vi "Analog Trigger.vi"() -> ()   [LabVIEW 2012]
uses:
  <vilib>/Platform/TimedLoop/XDataNode/timing_clust.ctl
  <vilib>/Platform/TimedLoop/XDataNode/nitl_modes.ctl
  <vilib>/Platform/TimedLoop/XDataNode/wakeup.ctl
  <vilib>/rvi/eio/common/nirviEmuTemplateMethod_errors.vi
  <vilib>/rvi/Emulation/niFpgaSctlEmulationRegisterWithScheduler.vi
  <vilib>/rvi/Emulation/niFpgaSctlEmulationScheduler.vi
  <vilib>/Platform/TimedLoop/XDataNode/XDataNode.xnode
  <vilib>/eio/EIONode/EIONode.xnode
  <vilib>/Platform/TimedLoop/XDataNode/XDNodeRunTimeDep.lvlib
panel:
  out "Over Threshold":bool
  in  "stop":bool
  in  "Threshold":i16
  out "AI Ch 0":i16
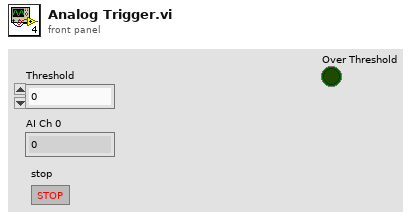
[diagram p1: front panel]
types:
  T1 = typedef "XDNodeRunTimeDep.lvlib/timing_clust.ctl" = cluster{"Expected End [f-1]":u64, "Actual End [f-1]":u64, "Finished Late? [f-1]":bool, "Expected End [i-1]":u64, "Actual End [i-1]":u64, "Finished Late? [i-1]":bool, "Expected Start [i]":u64, "Actual Start [i]":u64, "Expected Start [f]":u64, "Actual Start [f]":u64, "Source Name":string, "Structure Name":string, "Period":i64, "Deadline":i64, "Offset":i64, "Start":i64, "Priority":i32, "Timeout":i32, "Mode":T2, "Wakeup Reason":T3, "Error":errorcluster, "Source Type":string, "Secondary Source Type":string, "Global End Time":u64, "Global Start Time":u64, "Frame Duration":u64, "Iteration Duration":u64, "Assigned CPU":i32, "I/O Scan Engine Mode":u32}
  T2 = typedef "XDNodeRunTimeDep.lvlib/nitl_modes.ctl" = enum32{"No Change", "Process missed periods, maintain original phase", "Discard missed periods, maintain original phase", "Process missed periods, ignore original phase", "Discard missed periods, ignore original phase"}
  T3 = typedef "XDNodeRunTimeDep.lvlib/wakeup.ctl" = enum32{"Normal", "Aborted", "Asynchronous wakeup", "Timing source error", "Timed loop error", "Timeout"}
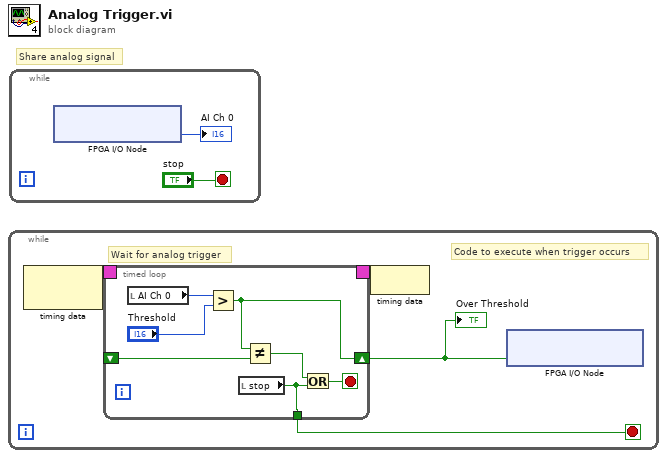
[diagram p0: block diagram]
diagram:
  # "Share analog signal"
  n1 = while {
    stop <- w1 stop-if-true
    # "Code to execute when trigger occurs"
    # "Wait for analog trigger"
    n2 = node-c288() -> (w4:T1)  [unwired: 1 in]
    n3 = timed-loop {
      timing: w4 -> [_]
      timing-out: [_] -> w3
      shift-right: [w9] -> w2
      shift-left: _ -> [w8]
      tunnel: [w5] -> w1
      stop <- w6 stop-if-true
      n4 = local read "AI Ch 0"() -> (w11:i16)
      n5 = Greater?(x=w11, y="Threshold") -> (0:w9:bool)
      n6 = local read "stop"() -> (w5:bool)
      n7 = Not Equal?(x=w9, y=w8) -> (x != y?=w7:bool)
      n8 = Or(x=w7, y=w5) -> (x .or. y?=w6:bool)
    }
    "Over Threshold" <- w2
    n9 = node-c288(w3) -> ()
    n10 = xnode "FPGA I/O Node"("Connector0/DIO0"=w2) -> ()  [unwired: 1 in, 1 out]
  }
  n11 = while {
    stop <- "stop" stop-if-true
    n12 = xnode "FPGA I/O Node"() -> ("Connector0/AI0"=→"AI Ch 0":i16)  [unwired: 1 in, 1 out]
  }
